vi "Impedance_Multi.vi"() -> ()   [LabVIEW 2021]
uses:
  <vilib>/DAQmx/write.llb/DAQmx Write (Analog Wfm 1Chan NSamp).vi
  <vilib>/DAQmx/read.llb/DAQmx Read (Analog 1D Wfm NChan NSamp).vi
  <vilib>/DAQmx/create/channels.llb/DAQmx Create Channel (AO-Voltage-Basic).vi
  <vilib>/DAQmx/configure/timing.llb/DAQmx Timing (Sample Clock).vi
  <vilib>/DAQmx/create/channels.llb/DAQmx Create Channel (AI-Voltage-Basic).vi
  <vilib>/DAQmx/miscellaneous.llb/DAQmx Fill In Error Info.vi
  <vilib>/DAQmx/configure/trigger.llb/DAQmx Start Trigger (Digital Edge).vi
  <vilib>/measure/maspectr.llb/FFT Spectrum (Mag-Phase) for N Chan.vi
  <vilib>/measure/matone.llb/Extract Single Tone Information N Chan.vi
  <vilib>/measure/NI_MABase.lvlib
  <vilib>/measure/NI_MAPro.lvlib
panel:
  in  "stop":bool
  out "Waveform sending":waveform(dbl)(graph)
  out "Residual":dbl[](graph)
  out "detected phases (deg)":dbl[](array[numeric]) format="%.2p"
  out "detected amplitudes":dbl[](array[numeric]) format="%.2p"
  out "detected frequencies":dbl[](array[numeric]) format="%.2p"
  out "FFT":cluster{"f0":dbl, "df":dbl, "magnitude":dbl[]}[](graph)
  out "Time domain":waveform(dbl)[](graph)
  in  "physical channels":tag
  out "data":waveform(dbl)[](array[waveform])
  in  "physical channels 2":tag
  in  "Time":dbl format="%#_6p"
  in  "amplitude":dbl=1.0 format="%0.2p"
  in  "frequency":dbl=10.0 format="%0.2p"
  in  "SampRate":dbl=1000.0 format="%0.2f"
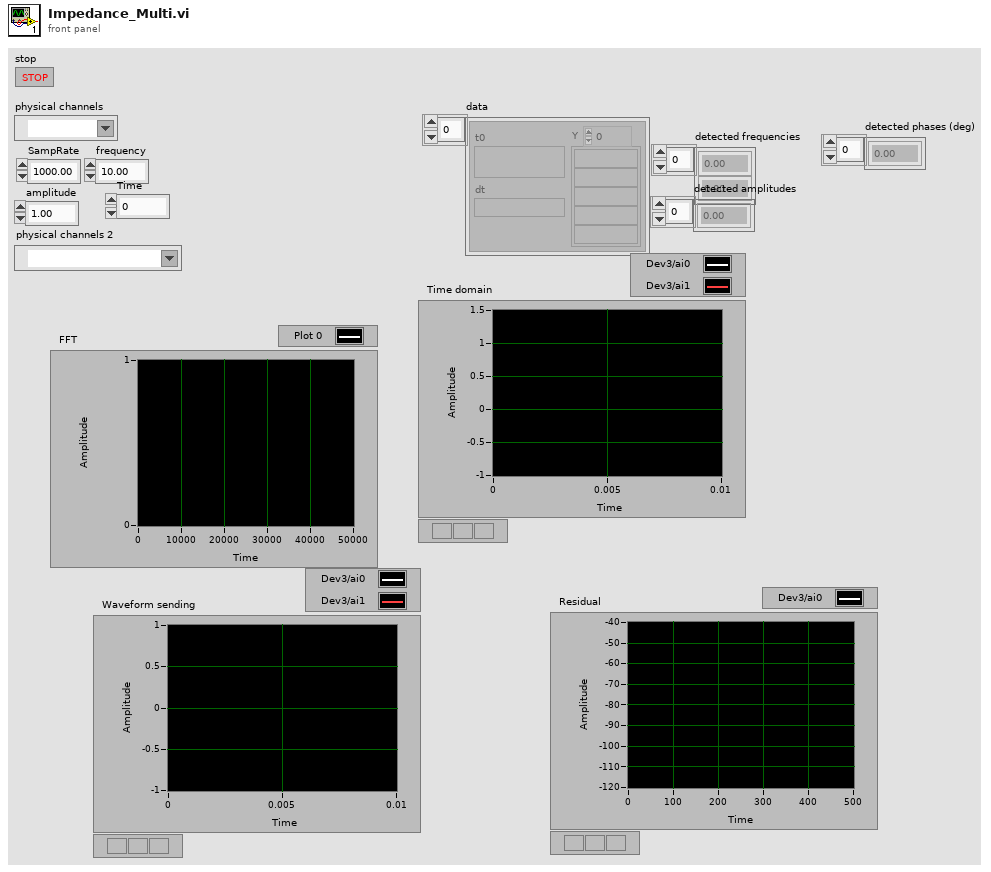
[diagram p1: front panel]
types:
  T1 = cluster{"approx freq. (optional)":dbl, "search (+/- % of Fsampl.)":dbl}
  T2 = enum32{"none", "input signal", "detected signal", "residual signal"}
  T3 = cluster{"exported time signal":waveform(dbl), "exported spectrum (dB)":cluster{"f0":dbl, "df":dbl, "dB Spectrum (Hann)":dbl[]}}[]
  T4 = cluster{"exported time signal":waveform(dbl), "exported spectrum (dB)":cluster{"f0":dbl, "df":dbl, "dB Spectrum (Hann)":dbl[]}}
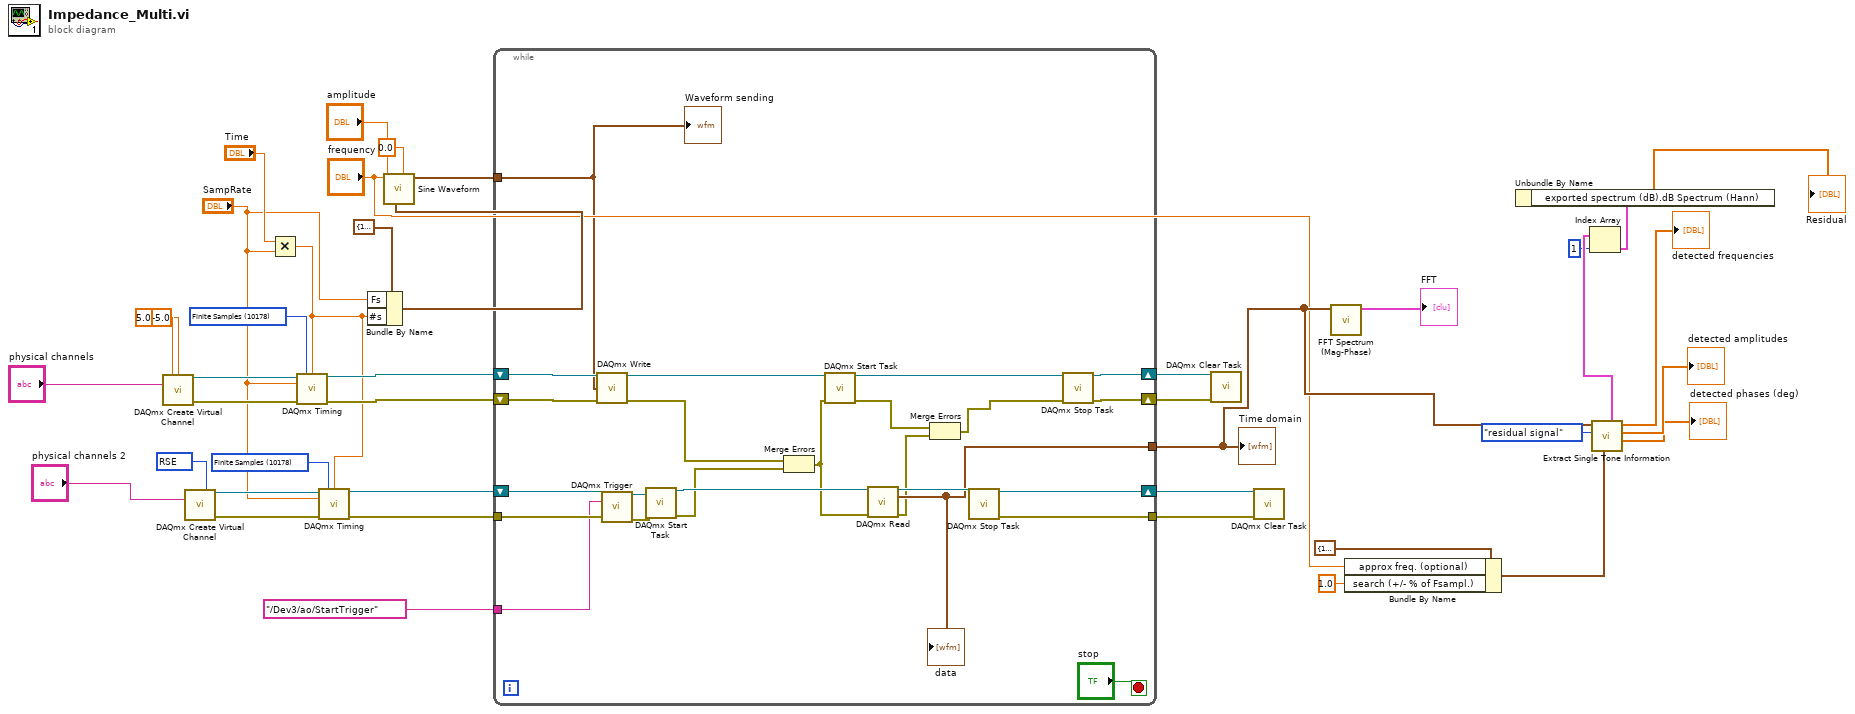
[diagram p0: block diagram]
diagram:
  w17 = 10083 items=["Default"=-1, "RSE"=10083, "NRSE"=10078, "Differential"=10106, "Pseudodifferential"=12529] ("input terminal configuration")
  w28 = 10178 items=["Finite Samples"=10178, "Continuous Samples"=10123, "Hardware Timed Single Point"=12522] ("sample mode")
  w32 = 10178 items=["Finite Samples"=10178, "Continuous Samples"=10123, "Hardware Timed Single Point"=12522] ("sample mode")
  n1 = call-poly <vilib>:"DAQmx Create Virtual Channel.vi"("maximum value"=5.0, "minimum value"=-5.0, "physical channels"="physical channels") -> ("task out"=w40:refnum<k21>, "error out"=w35:errorcluster)  [unwired: 11 in]
  n2 = call-poly <vilib>:"DAQmx Create Virtual Channel.vi"("input terminal configuration"=w17, "physical channels"="physical channels 2") -> ("task out"=w30:refnum<k21>, "error out"=w31:errorcluster)  [unwired: 12 in]
  n3 = Multiply(x="Time", y="SampRate") -> (x*y=w20:dbl)
  n4 = call-poly <vilib>:"DAQmx Timing.vi"("task/channels in"=w40, "sample mode"=w32, "samples per channel"=w20, "rate"="SampRate", "error in"=w35) -> ("task out"=w39:refnum<k21>, "error out"=w36:errorcluster)  [unwired: 9 in]
  n5 = call-poly <vilib>:"DAQmx Timing.vi"("task/channels in"=w30, "sample mode"=w28, "samples per channel"=w20, "rate"="SampRate", "error in"=w31) -> ("task out"=w27:refnum<k21>, "error out"=w26:errorcluster)  [unwired: 9 in]
  n6 = Bundle By Name(cluster=cluster{"Fs":dbl, "#s":dbl} {"Fs"=1000.0, "#s"=1000.0} ("sampling info"), "Fs"="SampRate", "#s"=w20) -> (w19:cluster{"Fs":dbl, "#s":dbl})
  n7 = call <vilib>:"Sine Waveform.vi"("offset"=0.0, "sampling info"=w19, "amplitude"="amplitude", "frequency"="frequency") -> ("signal out"=w6:waveform(dbl))  [unwired: 6 in, 1 out]
  n8 = while {
    tunnel: w26 -> [w60]
    tunnel: [w56] -> w25
    tunnel: tag "/Dev3/ao/StartTrigger" ("source") -> [w50]
    tunnel: [w49] -> w15
    tunnel: w6 -> [w48]
    shift-right: [w62] -> w34
    shift-left: w39 -> [w66]
    shift-right: [w47] -> w5
    shift-left: w36 -> [w64]
    shift-right: [w55] -> w24
    shift-left: w27 -> [w61]
    stop <- "stop" stop-if-true
    n9 = call-poly <vilib>:"DAQmx Write.vi"("task/channels in"=w66, "data"=w48, "error in"=w64) -> ("task out"=w65:refnum<k21>, "error out"=w52:errorcluster)  [unwired: 10 in, 1 out]
    n10 = call-poly <vilib>:"DAQmx Trigger.vi"("task/channels in"=w61, "source"=w50, "error in"=w60) -> ("task out"=w58:refnum<k21>, "error out"=w59:errorcluster)  [unwired: 11 in]
    n11 = call <vilib>:"DAQmx Start Task.vi"("task/channels in"=w58, "error in"=w59) -> ("task out"=w57:refnum<k21>, "error out"=w53:errorcluster)  [unwired: 12 in]
    n12 = Merge Errors(w52, w53) -> (w51:errorcluster)
    n13 = call <vilib>:"DAQmx Start Task.vi"("task/channels in"=w65, "error in"=w51) -> ("task out"=w63:refnum<k21>, "error out"=w45:errorcluster)  [unwired: 12 in]
    n14 = call-poly <vilib>:"DAQmx Read.vi"("task/channels in"=w57, "error in"=w51) -> ("task out"=w54:refnum<k21>, "data"=w49:waveform(dbl)[], "error out"=w46:errorcluster)  [unwired: 11 in]
    "data" <- w49
    n15 = Merge Errors(w45, w46) -> (w44:errorcluster)
    n16 = call <vilib>:"DAQmx Stop Task.vi"("task/channels in"=w54) -> ("task out"=w55:refnum<k21>, "error out"=w56:errorcluster)  [unwired: 13 in]
    n17 = call <vilib>:"DAQmx Stop Task.vi"("task/channels in"=w63, "error in"=w44) -> ("task out"=w62:refnum<k21>, "error out"=w47:errorcluster)  [unwired: 12 in]
    "Waveform sending" <- w48
  }
  "Time domain" <- w15
  n18 = call <vilib>:"DAQmx Clear Task.vi"("task in"=w34, "error in"=w5) -> ()  [unwired: 13 in, 1 out]
  n19 = call <vilib>:"DAQmx Clear Task.vi"("task in"=w24, "error in"=w25) -> ()  [unwired: 13 in, 1 out]
  n20 = call-poly <vilib>:"FFT Spectrum (Mag-Phase).vi"("time signals"=w15) -> ("magnitudes"=→"FFT":cluster{"f0":dbl, "df":dbl, "magnitude":dbl[]}[])  [unwired: 6 in, 4 out]
  n21 = Bundle By Name(cluster=T1 {"approx freq. (optional)"=100.0, "search (+/- % of Fsampl.)"=0.0} ("advanced search"), "approx freq. (optional)"="frequency", "search (+/- % of Fsampl.)"=1.0) -> (w2:T1)
  n22 = call-poly <vilib>:"Extract Single Tone Information.vi"("advanced search"=w2, "export mode"=T2."residual signal", "time signals in"=w15) -> ("detected phases (deg)"=→"detected phases (deg)":dbl[], "detected amplitudes"=→"detected amplitudes":dbl[], "detected frequencies"=→"detected frequencies":dbl[], "exported signals"=w10:T3)  [unwired: 3 in, 2 out]
  n23 = Index Array(array=w10, index=1) -> (element=w8:T4)
  n24 = Unbundle By Name(w8) -> ("exported spectrum (dB).dB Spectrum (Hann)"=→"Residual":dbl[])
